vi "Attente retour autotest.vi"(8 "error in (no error)":errorcluster caption="entrée d'erreur (pas d'erreur)", 9 "Realize Autotest ?":bool=TRUE, 10 "Type Product":string(combo)="PCBA", 11 "Part Number PCBA":string(combo)) -> (0 "error out":errorcluster caption="sortie d'erreur", 3 "Autotest OK":bool)   [LabVIEW 2020]
uses:
  Class/Popup/Popup Autotest_With_Actor/Popup Autotest_With_Actor.lvclass
  C:/Users/ngarcin/OneDrive - Altyor/Standard TB/Class/Popup/Class Popup Autotest (Default)/Popup Autotest (Default).lvclass
  C:/Users/ngarcin/OneDrive - Altyor/Standard TB/Class/Popup/Class Popup (Main)/Class Popup (Main).lvclass
  Class/Popup/Popup Autotest_Without_Actor/Popup Autotest_Without_Actor.lvclass
  Class/Instrument/Instrument (Default)/Class Instrument (Default).lvclass
  Commun VI/Library Commun.lvlib
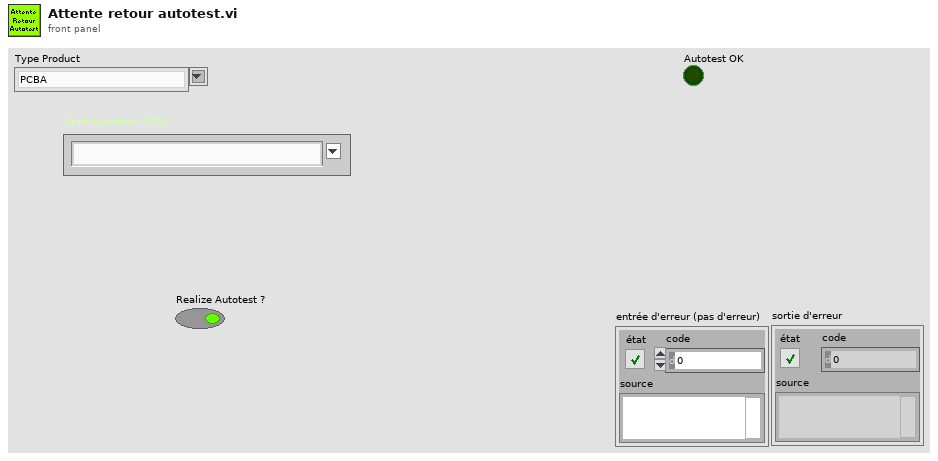
[diagram p1: front panel]
types:
  T1 = enum16{"Add Instr", "Remove Instr", "List Instr", "Get Instr Class", "Get Instr obj", "Save Insrt obj", "Modify Insrt obj", "Init"}
  T2 = cluster{"Name":string, "Instrument":refnum<class "Class Instrument (Default).lvclass">, "Close After Autotest":bool}[]
  T3 = cluster{"Name":string, "Instrument":refnum<class "Class Instrument (Default).lvclass">, "Close After Autotest":bool}
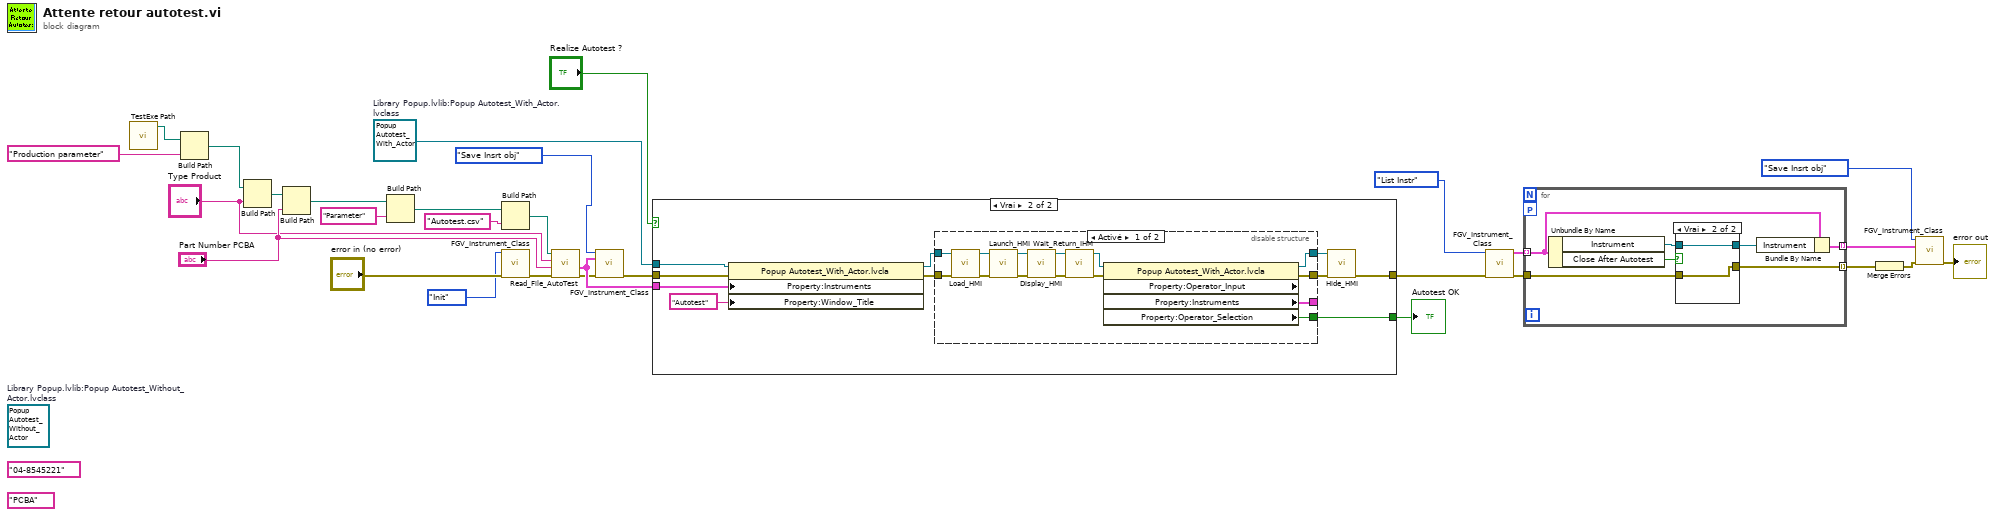
[diagram p0: block diagram]
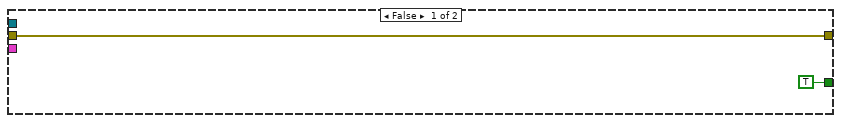
[diagram p2: hidden frame]
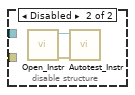
[diagram p3: hidden frame]
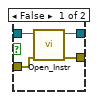
[diagram p4: hidden frame]
diagram:
  w5 = refnum<class "Popup Autotest_With_Actor.lvclass"> refnum  # Library Popup.lvlib:Popup Autotest_With_Actor.lvclass
  (unwired) "04-8545221" ("Part Number PCBA")
  (unwired) "PCBA" ("Type Product")
  (unwired) refnum<class "Popup Autotest_Without_Actor.lvclass"> refnum  # Library Popup.lvlib:Popup Autotest_Without_Actor.lvclass
  n1 = call "TestExe Path.vi"() -> ("Chemin Actuel"=w29:path)  [unwired: 9 in, 2 out]
  n2 = Build Path(base path=w29, name or relative path="Production parameter" ("nom ou chemin relatif")) -> (appended path=w28:path)
  n3 = Build Path(base path=w28, name or relative path="Type Product") -> (appended path=w27:path)
  n4 = Build Path(base path=w27, name or relative path="Part Number PCBA") -> (appended path=w26:path)
  n5 = Build Path(base path=w26, name or relative path="Parameter" ("nom ou chemin relatif")) -> (appended path=w24:path)
  n6 = Build Path(base path=w24, name or relative path="Autotest.csv" ("nom ou chemin relatif")) -> (appended path=w23:path)
  n7 = call "FGV_Instrument_Class.vi"("Action"=T1."Init", "error in (no error)"="error in (no error)") -> ("error out"=w13:errorcluster)  [unwired: 11 in, 2 out]
  n8 = call "Read_File_AutoTest.vi"("error in"=w13, "Part Number PCBA"="Part Number PCBA", "Type Product"="Type Product", "file path"=w23) -> ("error out"=w20:errorcluster, "Instruments"=w21:T2)  [unwired: 4 in, 2 out]
  n9 = call "FGV_Instrument_Class.vi"("Action"=T1."Save Insrt obj", "Instruments"=w21, "error in (no error)"=w20) -> ("error out"=w19:errorcluster)  [unwired: 10 in, 2 out]
  n10 = case shown="Vrai" "Realize Autotest ?" {
    tunnel: w5 -> [_ w38]
    tunnel: w21 -> [_ w36]
    tunnel: w19 -> [w32 w35]
    tunnel: [w32 w34] -> w18
    tunnel: [TRUE ("Property:Operator_Selection") w33] -> w9
    frame False {
    }
    frame True {
      n11 = property class="Popup Autotest_With_Actor.lvcla"(reference=w38, error in=w35, "Property:Instruments"=w36, "Property:Window_Title"="Autotest" ("Window_Title")) -> (reference out=w42:refnum<class "Popup Autotest_With_Actor.lvclass">, error out=w41:errorcluster)
      n12 = disable-structure shown="Activé" {
        disable-tunnel: w42 -> [w50 _]
        disable-tunnel: w41 -> [w49 _]
        disable-tunnel: [w46 _] -> w40
        disable-tunnel: [w45 _] -> w39
        disable-tunnel: [w44 _] -> _
        disable-tunnel: [w43 _] -> w33
        frame Enabled {
          n13 = call-dynamic "Load_HMI.vi"("error in (no error)"=w49, "Class Popup (Default) en entrée"=w50) -> ("error out"=w56:errorcluster, "Class Popup (Default) en sortie"=w55:refnum<class "Popup Autotest_With_Actor.lvclass">)  [unwired: 8 in]
          n14 = call-dynamic "Launch_HMI.vi"("error in (no error)"=w56, "Class Popup (Default) en entrée"=w55) -> ("error out"=w54:errorcluster, "Class Popup (Default) en sortie"=w52:refnum<class "Popup Autotest_With_Actor.lvclass">)  [unwired: 8 in]
          n15 = call-dynamic "Display_HMI.vi"("error in (no error)"=w54, "Class Popup (Default) en entrée"=w52) -> ("error out"=w53:errorcluster, "Class Popup (Default) en sortie"=w51:refnum<class "Popup Autotest_With_Actor.lvclass">)  [unwired: 8 in]
          n16 = call-dynamic "Wait_Return_IHM.vi"("error in (no error)"=w53, "Class Popup (Default) en entrée"=w51) -> ("error out"=w47:errorcluster, "Class Popup (Default) en sortie"=w48:refnum<class "Popup Autotest_With_Actor.lvclass">)  [unwired: 8 in]
          n17 = property class="Popup Autotest_With_Actor.lvcla" props=["Property:Operator_Input", "Property:Instruments", "Property:Operator_Selection"](reference=w48, error in=w47) -> (reference out=w46:refnum<class "Popup Autotest_With_Actor.lvclass">, error out=w45:errorcluster, "Property:Instruments"=w44:T2, "Property:Operator_Selection"=w43:bool)  [unwired: 1 out]
        }
        frame Disabled {
          n18 = call-dynamic "Open_Instr.vi"() -> ("error out"=w57:errorcluster, "Class Multimeter (Default) en sortie"=w58:refnum<class "Class Instrument (Default).lvclass">)  [unwired: 10 in]
          n19 = call-dynamic "Autotest_Instr.vi"("error in (no error)"=w57, "Class Instrument (Default) en entrée"=w58) -> ()  [unwired: 8 in, 2 out]
        }
      }
      n20 = call-dynamic "Hide_HMI.vi"("error in (no error)"=w39, "Class Popup (Default) en entrée"=w40) -> ("error out"=w34:errorcluster)  [unwired: 8 in, 1 out]
    }
  }
  "Autotest OK" <- w9
  n21 = call "FGV_Instrument_Class.vi"("Action"=T1."List Instr", "error in (no error)"=w18) -> ("Instruments 2"=w17:T2, "error out"=w8:errorcluster)  [unwired: 11 in, 1 out]
  n22 = for {
    tunnel: w17 -> [w64] mode=indexing
    tunnel: [w62] -> w15 mode=indexing
    workers-P: _ -> [_]
    tunnel: w8 -> [w61]
    tunnel: [w60] -> w7 mode=indexing
    n23 = Unbundle By Name(w64) -> ("Instrument"=w65:refnum<class "Class Instrument (Default).lvclass">, "Close After Autotest"=w59:bool)
    n24 = case shown="Vrai" w59 {
      tunnel: w65 -> [w69 w71]
      tunnel: [w68 w71] -> w63
      tunnel: w61 -> [w67 w70]
      tunnel: [w66 w70] -> w60
      frame False {
        n25 = call-dynamic "Open_Instr.vi"("error in (no error)"=w67, "Class Multimeter (Default) en entrée"=w69) -> ("error out"=w66:errorcluster, "Class Multimeter (Default) en sortie"=w68:refnum<class "Class Instrument (Default).lvclass">)  [unwired: 8 in]
      }
      frame True {
      }
    }
    n26 = Bundle By Name(cluster=w64, "Instrument"=w63) -> (w62:T3)
  }
  n27 = Merge Errors(w7) -> (w6:errorcluster)
  n28 = call "FGV_Instrument_Class.vi"("Action"=T1."Save Insrt obj", "Instruments"=w15, "error in (no error)"=w6) -> ("error out"=→"error out":errorcluster)  [unwired: 10 in, 2 out]
